vi "subvi_Numbering_Set_CH_Indicator.vi"(8 "# of Channel":i32, 9 "# of Set":i32, 10 "CH data":i32, 11 "Set data":i32) -> (0 "CH state":string, 1 "CH value":i32, 2 "Set state":string, 3 "Set value":i32)   [LabVIEW 2016]
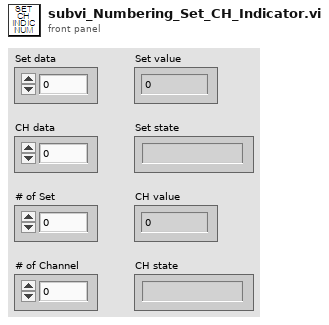
[diagram p1: front panel]
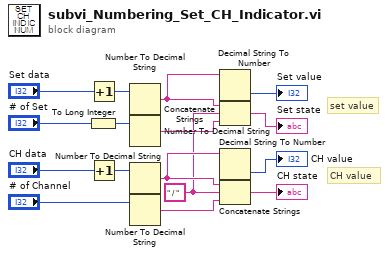
[diagram p0: block diagram]
diagram:
  w1 = " / " ("문자열")
  # "CH value"
  # "set value"
  n1 = To Long Integer(number="# of Set") -> (32bit integer=w12:i32)
  n2 = Increment(x="Set data") -> (x+1=w3:i32)
  n3 = Increment(x="CH data") -> (x+1=w8:i32)
  n4 = Number To Decimal String(number=w3) -> (decimal integer string=w13:string)  [unwired: 1 in]
  n5 = Number To Decimal String(number=w12) -> (decimal integer string=w4:string)  [unwired: 1 in]
  n6 = Number To Decimal String(number=w8) -> (decimal integer string=w14:string)  [unwired: 1 in]
  n7 = Number To Decimal String(number="# of Channel") -> (decimal integer string=w6:string)  [unwired: 1 in]
  n8 = Decimal String To Number(string=w13) -> (number=→"Set value":i32)  [unwired: 2 in, 1 out]
  n9 = Concatenate Strings(w13, w1, w4) -> (→"Set state":string)
  n10 = Decimal String To Number(string=w14) -> (number=→"CH value":i32)  [unwired: 2 in, 1 out]
  n11 = Concatenate Strings(w14, w1, w6) -> (→"CH state":string)
